vi "Material-ConfigDialog-Construct.vi"(11 "error in":errorcluster) -> (4 "Configuration Dialog":refnum<class "Material-ConfigDialog.lvclass">, 6 "Configuration Dialog Mailbox":refnum<event-registration>, 15 "error out":errorcluster)   [LabVIEW 2013, in "Material-ConfigDialog.lvclass"]
uses:
  Material-ConfigDialog.lvclass
  Reuse Library/featherweight/Core/Messaging/Message/FTW-Message.lvclass
  Reuse Library/featherweight/Core/Messaging/Messenger.Actor/FTW-Messenger-Actor.lvclass
  Material-ConfigDialog.lvclass/Material-ConfigDialog.ctl
  Reuse Library/featherweight/Core/Messaging/Messenger/FTW-Messenger.lvclass
panel:
  # "Inputs"
  # "Outputs"
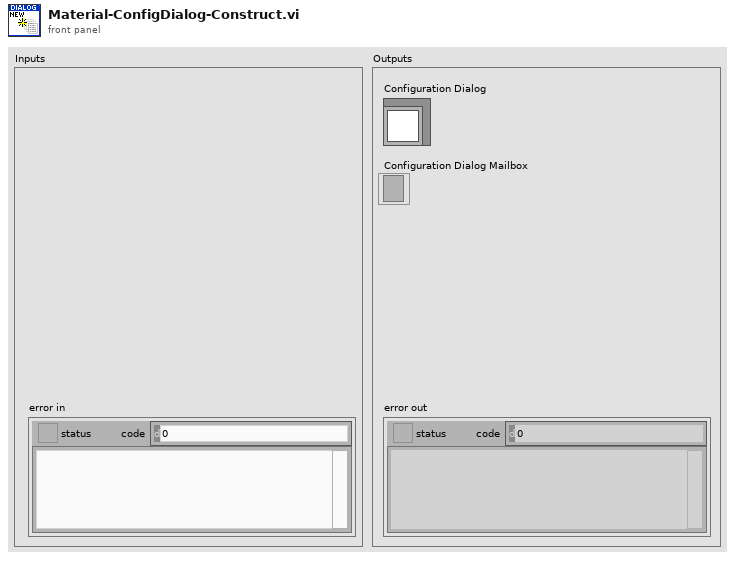
[diagram p1: front panel]
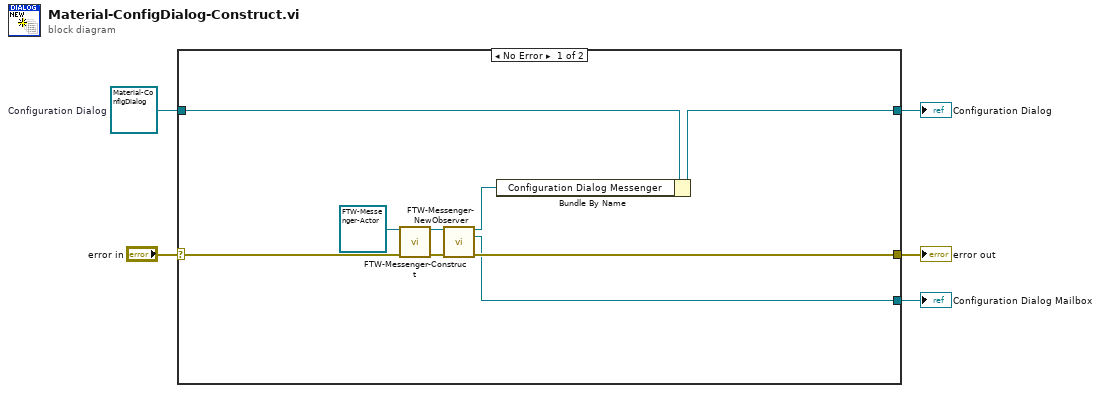
[diagram p0: block diagram]
diagram:
  w4 = refnum<class "Material-ConfigDialog.lvclass"> refnum  # Configuration Dialog
  n1 = case shown="No Error" "error in" {
    selector: "error in" -> [w6 w16]
    tunnel: [w10 w16] -> w5
    tunnel: [w13 w15] -> w3
    tunnel: w4 -> [w14 w15]
    tunnel: [w8 _] -> w1
    frame No Error {
      n2 = call-dynamic "FTW-Messenger-Construct.vi"("Messenger Type"=refnum<class "FTW-Messenger-Actor.lvclass"> refnum, "error in"=w6) -> ("Actor Messenger"=w12:refnum<class "FTW-Messenger-Actor.lvclass">, "error out"=w11:errorcluster)  [unwired: 12 in]
      n3 = call "FTW-Messenger-NewObserver.vi"("Messenger"=w12, "error in"=w11) -> ("Messenger out"=w9:refnum<class "FTW-Messenger-Actor.lvclass">, "Message"=w8:refnum<event-registration>, "error out"=w10:errorcluster)  [unwired: 11 in]
      n4 = Bundle By Name(cluster=w14, "Configuration Dialog Messenger"=w9) -> (w13:refnum<class "Material-ConfigDialog.lvclass">)
    }
    frame Error {
    }
  }
  "error out" <- w5
  "Configuration Dialog" <- w3
  "Configuration Dialog Mailbox" <- w1
